vi "Get Request Type.vi"(8 "error in (no error)":errorcluster, 11 "SetInputMute in":refnum<class "SetInputMute.lvclass">) -> (0 "error out":errorcluster, 2 "Request Type":string, 3 "SetInputMute out":refnum<class "SetInputMute.lvclass">)   [LabVIEW 2020, in "obs-websocket.lvlib" / "SetInputMute.lvclass"]
uses:
  SetInputMute.lvclass
  SetInputMute.lvclass/SetInputMute.ctl
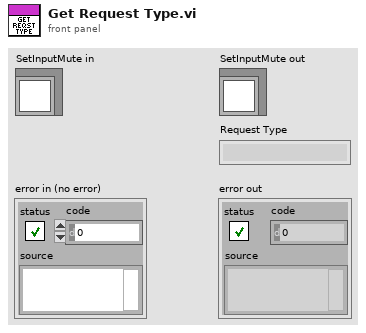
[diagram p1: front panel]
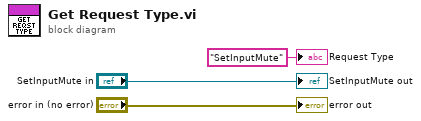
[diagram p0: block diagram]
diagram:
  "error out" <- "error in (no error)"
  "SetInputMute out" <- "SetInputMute in"
  "Request Type" <- "SetInputMute" ("Request Type")
